vi "Read ADU Packet.vi"(8 "error in":errorcluster, 10 "isMaster (f)":bool, 11 "IP transmission data unit in":refnum<class "IP Data Unit.lvclass">) -> (0 "error out":errorcluster, 1 "modbus data unit":refnum<class "Modbus Data Unit.lvclass">, 3 "IP transmission data unit out":refnum<class "IP Data Unit.lvclass">, 5 "PDU Valid?":bool)   [LabVIEW 2021, in "IP Data Unit.lvclass"]
doc: "This uses the protocol layer to read a modbus packet off of the bus, wrapped in the IP transmission data unit."
uses:
  IP Data Unit.lvclass
  D:/my_projects/projects/Algorithms/Labview/21/Modbus_v121c/Transmission Data Unit/Transmission Data Unit.lvclass
  Modbus Data Unit/Modbus Data Unit.lvclass
  IP Data Unit.lvclass/IP Data Unit.ctl
  Transmission Data Unit.lvclass/Transmission Data Unit.ctl
  Modbus Data Unit/Modbus Data Unit.lvclass/Modbus Data Unit.ctl
  <vilib>/Utility/error.llb/Clear Errors.vi
  Transmission Data Unit.lvclass
  Network Interface/TCP Interface/TCP Shared Components/TCP Shared Components.lvlib
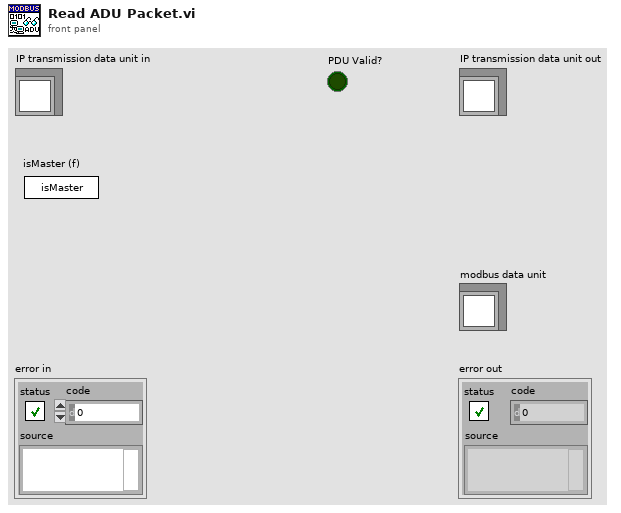
[diagram p1: front panel]
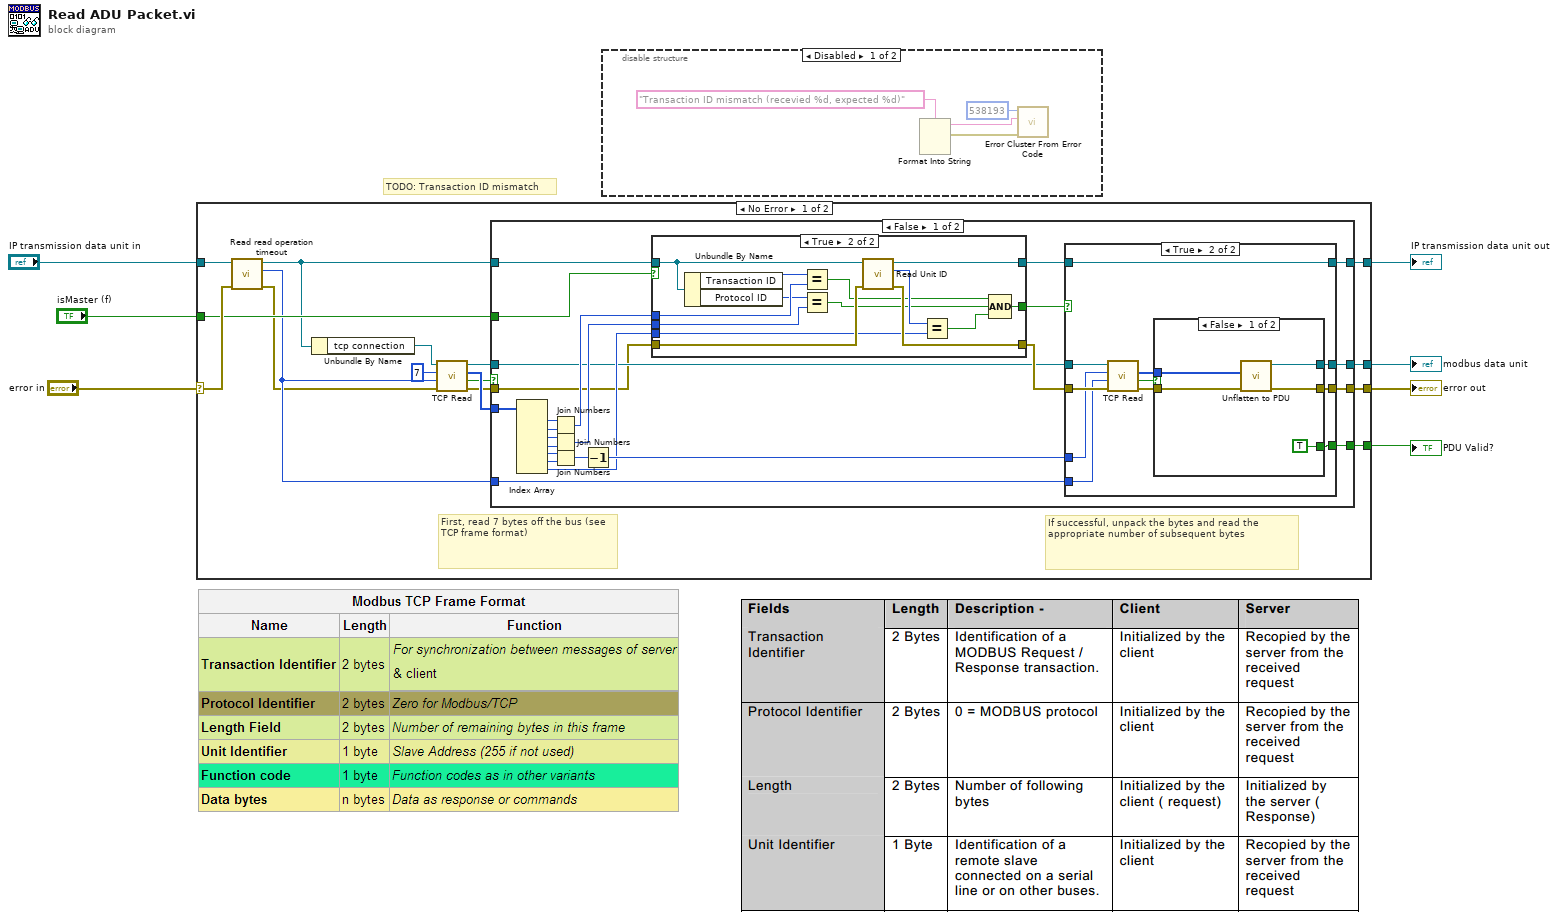
[diagram p0: block diagram]
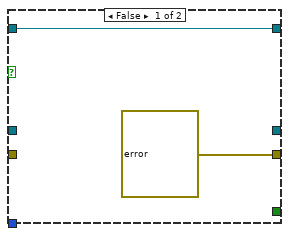
[diagram p2: hidden frame]
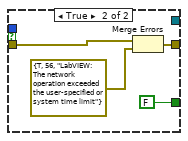
[diagram p3: hidden frame]
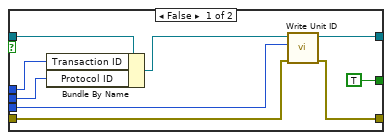
[diagram p4: hidden frame]
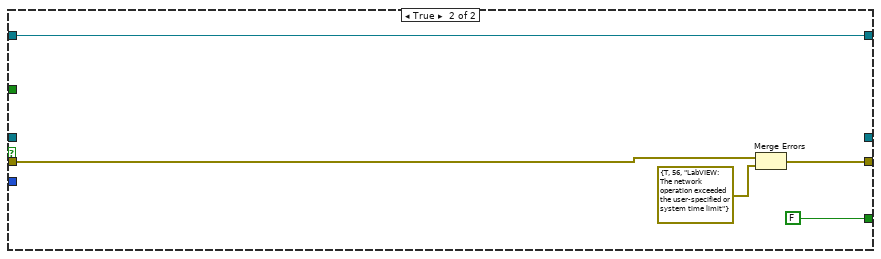
[diagram p5: hidden frame]
diagram:
  # "TODO: Transaction ID mismatch"
  n1 = case shown="No Error" "error in" {
    selector: "error in" -> [w19 w99]
    tunnel: [w22 w99] -> w3
    tunnel: "IP transmission data unit in" -> [w20 w98]
    tunnel: [w23 w98] -> w6
    tunnel: [w21 _] -> w5
    tunnel: [w18 _] -> w4
    tunnel: "isMaster (f)" -> [w17 _]
    frame No Error {
      # "If successful, unpack the bytes and read the appropriate number of subsequent bytes"
      # "First, read 7 bytes off the bus (see TCP frame format)"
      n2 = call "Read read operation timeout.vi"("error in (no error)"=w19, "transmission data unit in"=w20) -> ("error out"=w8:errorcluster, "read operation timeout"=w11:i32, "transmission data unit out"=w9:refnum<class "IP Data Unit.lvclass">)  [unwired: 7 in]
      n3 = Unbundle By Name(w9) -> ("tcp connection"=w16:refnum<k5>)
      n4 = call "TCP Read.vi"("error in"=w8, "timeout"=w11, "bytes to read"=7 ("Bytes to Read"), "connection ID"=w16) -> ("error out"=w12:errorcluster, "timed out?"=w13:bool, "data"=w14:u8[], "connection ID out"=w10:refnum<k5>)  [unwired: 4 in]
      n5 = case shown="False" w13 {
        tunnel: w14 -> [w47 _]
        tunnel: w9 -> [w32 w97]
        tunnel: [w35 w97] -> w23
        tunnel: w10 -> [w25 _]
        tunnel: w11 -> [w39 _]
        tunnel: w12 -> [w24 w95]
        tunnel: [w37 w96] -> w22
        tunnel: [w36 _] -> w21
        tunnel: [w34 FALSE] -> w18
        tunnel: w17 -> [w26 _]
        frame False {
          n6 = Index Array(array=w47) -> (element #1=w45:u8, element #2=w46:u8, element #3=w44:u8, element #4=w43:u8, element #5=w41:u8, element #6=w42:u8, element #7=w28:u8)  [unwired: 7 in]
          n7 = Join Numbers(hi=w45, lo=w46) -> ((hi.lo)=w33:u16)
          n8 = Join Numbers(hi=w44, lo=w43) -> ((hi.lo)=w30:u16)
          n9 = Join Numbers(hi=w41, lo=w42) -> ((hi.lo)=w40:u16)
          n10 = Decrement(x=w40) -> (x-1=w38:u16)
          n11 = case shown="True" w26 {
            tunnel: w32 -> [w78 w83]
            tunnel: w33 -> [w77 w92]
            tunnel: [TRUE w87] -> w31
            tunnel: [w75 w85] -> w27
            tunnel: w30 -> [w72 w84]
            tunnel: w24 -> [w71 w89]
            tunnel: [w74 w90] -> w29
            tunnel: w28 -> [w73 w88]
            frame False {
              n12 = Bundle By Name(cluster=w78, "Transaction ID"=w77, "Protocol ID"=w72) -> (w70:refnum<class "IP Data Unit.lvclass">)
              n13 = call "Write Unit ID.vi"("error in"=w71, "unit ID"=w73, "transmission data unit in"=w70) -> ("error out"=w74:errorcluster, "transmission data unit out"=w75:refnum<class "IP Data Unit.lvclass">)  [unwired: 7 in]
            }
            frame True {
              n14 = Unbundle By Name(w83) -> ("Transaction ID"=w82:u16, "Protocol ID"=w81:u16)
              n15 = Equal?(x=w82, y=w92) -> (x = y?=w86:bool)
              n16 = Equal?(x=w81, y=w84) -> (x = y?=w79:bool)
              n17 = call "Read Unit ID.vi"("error in"=w89, "transmission data unit in"=w83) -> ("error out"=w90:errorcluster, "unit ID"=w91:u8, "transmission data unit out"=w85:refnum<class "IP Data Unit.lvclass">)  [unwired: 7 in]
              n18 = Equal?(x=w91, y=w88) -> (x = y?=w80:bool)
              n19 = Compound Arithmetic op=AND(w86, w79, w80) -> (w87:bool)
            }
          }
          n20 = case shown="True" w31 {
            tunnel: w39 -> [_ w54]
            tunnel: w38 -> [_ w53]
            tunnel: [errorcluster {"status"=TRUE, "code"=-1967353903, "source"="LabVIEW DSC: The communication between the Modbus master and slave devices was interrupted. Check the connection status between the two devices."} ("error out") w60] -> w37
            tunnel: [_ w59] -> w36
            tunnel: w27 -> [w49 w57]
            tunnel: [w49 w57] -> w35
            tunnel: [_ w58] -> w34
            tunnel: w29 -> [_ w55]
            tunnel: w25 -> [_ w56]
            frame False {
            }
            frame True {
              n21 = call "TCP Read.vi"("error in"=w55, "timeout"=w54, "bytes to read"=w53, "connection ID"=w56) -> ("error out"=w52:errorcluster, "timed out?"=w51:bool, "data"=w50:u8[])  [unwired: 4 in, 1 out]
              n22 = case shown="False" w51 {
                tunnel: w52 -> [w64 w68]
                tunnel: [w63 w69] -> w60
                tunnel: [w61 _] -> w59
                tunnel: w50 -> [w62 _]
                tunnel: [TRUE FALSE] -> w58
                frame False {
                  n23 = call "Unflatten to PDU.vi"("error in"=w64, "modbus data unit data"=w62) -> ("error out"=w63:errorcluster, "modbus data unit out"=w61:refnum<class "Modbus Data Unit.lvclass">)  [unwired: 8 in]
                }
                frame True {
                  n24 = Merge Errors(w68, errorcluster {"status"=TRUE, "code"=56, "source"="LabVIEW: The network operation exceeded the user-specified or system time limit"} ("error out")) -> (w69:errorcluster)
                }
              }
            }
          }
        }
        frame True {
          n25 = Merge Errors(w95, errorcluster {"status"=TRUE, "code"=56, "source"="LabVIEW: The network operation exceeded the user-specified or system time limit"} ("error out")) -> (w96:errorcluster)
        }
      }
    }
    frame Error {
    }
  }
  "error out" <- w3
  "IP transmission data unit out" <- w6
  "modbus data unit" <- w5
  "PDU Valid?" <- w4
  n26 = disable-structure shown="Disabled" {
    frame Disabled {
      n27 = Format Into String(format string="Transaction ID mismatch (recevied %d, expected %d)") -> (resulting string=w103:string, error in=w105:errorcluster, error out=w104:errorcluster, w101:u16, w100:u16)  [unwired: 1 in]
      n28 = call <vilib>:"Error Cluster From Error Code.vi"("error in (no error)"=w104, "error message (\"\")"=w103, "error code (0)"=538193) -> ()  [unwired: 6 in, 1 out]
    }
    frame Enabled {
    }
  }
